vi "init.vi"(8 "error in (no error)":errorcluster, 11 "Soda Actor in":refnum<class "Soda Actor.lvclass">) -> (0 "error out":errorcluster, 3 "Soda Actor out":refnum<class "Soda Actor.lvclass">)   [LabVIEW 2019, in "Soda Actor.lvlib" / "Soda Actor.lvclass"]
uses:
  Soda Actor.lvclass
  Soda Actor.lvclass/Soda Actor.ctl
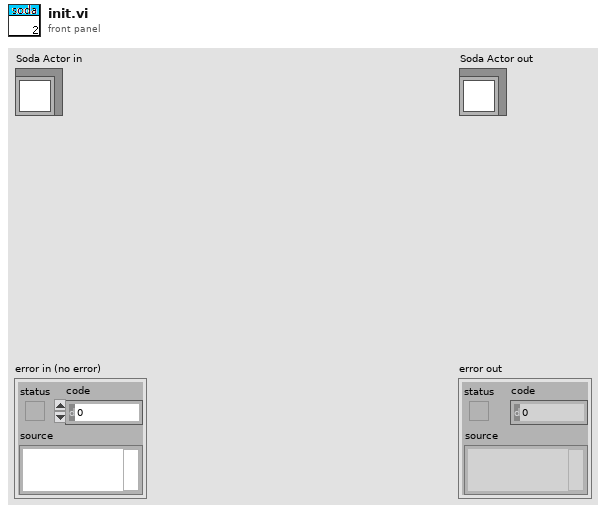
[diagram p1: front panel]
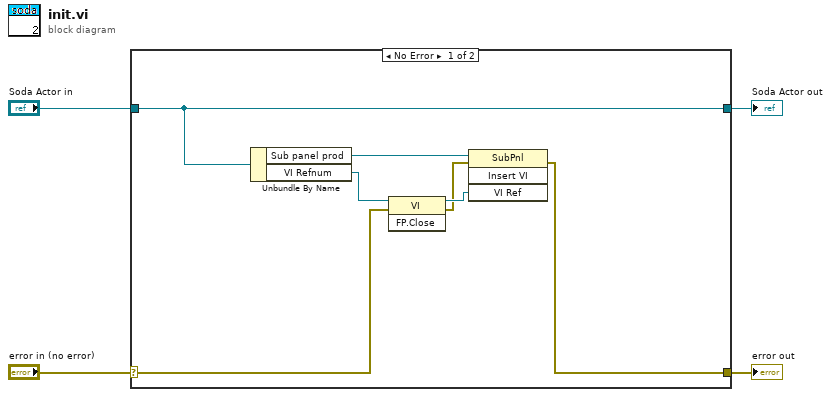
[diagram p0: block diagram]
diagram:
  n1 = case shown="No Error" "error in (no error)" {
    selector: "error in (no error)" -> [w9 w13]
    tunnel: [w5 w13] -> w3
    tunnel: [w10 w12] -> w1
    tunnel: "Soda Actor in" -> [w10 w12]
    frame No Error {
      n2 = Unbundle By Name(w10) -> ("Sub panel prod"=w7:refnum<vi>, "VI Refnum"=w8:refnum<vi>)
      n3 = invoke class="VI" method="FP.Close"(reference=w8, error in=w9) -> (reference out=w11:refnum<vi>, error out=w6:errorcluster)  [unwired: 1 in, 1 out]
      n4 = invoke class="SubPnl" method="Insert VI"(reference=w7, error in=w6, "VI Ref"=w11) -> (error out=w5:errorcluster)  [unwired: 1 in, 3 out]
    }
    frame Error {
    }
  }
  "error out" <- w3
  "Soda Actor out" <- w1
